vi "temp.vi"   [LabVIEW 2017]
uses:
  Configuration Database/Controls/Congif Data.ctl
  Configuration Database/Controls/Config Commands.ctl
  Error Handler/Controls/Error Type.ctl
  Error Handler/Controls/Error Data.ctl
  Views/Entry Console View/Controls/Entry Console Data.ctl
  Car Wash Controller/Controls/Car Wash States.ctl
  Car Wash Controller/Controls/Vehicle Location.ctl
  Car Wash Controller/Controls/Controller Overhead.ctl
  Car Wash Controller/Controls/CarWash CMD.ctl
  Views/Wash Display Console View/Controls/Car Wash Indicators.ctl
types:
  T1 = typedef "Car Wash Indicators.ctl" = cluster{"Under Body Wash":bool, "Bug Remover":bool, "Pre-Soak":bool, "High Pressure Wash":bool, "Low Pressure Wax":bool, "Spot Free Rinse":bool, "Tire Shine Foam":bool, "Air Dry":bool}
  T2 = typedef "CarWash CMD.ctl" = cluster{"CarWash States":T3, "Variant":variant}
  T3 = typedef "Car Wash States.ctl" = enum16{"Initial", "Wait for start", "Start", "Wait for vehicle", "Wash Step Execution", "Wash Step/Cycle Complete", "Wash Exit", "Wash Abort/Terminate"}
  T4 = typedef "Controller Overhead.ctl" = cluster{"Location change":bool, "Vehicle Location":T5, "CarWash State":T3, "CarWash Next State":T3, "Start change":bool, "Time":dbl, "Elapsed Time":dbl}
  T5 = typedef "Vehicle Location.ctl" = enum16{"Entry", "Station 1", "Station 2", "Station 3", "Exit"}
  T6 = typedef "Car Wash States.ctl" = enum16{"Initial", "Wait for start", "Start", "Wait for vehicle", "Wash Step Execution", "Wash Step Complete", "Wash Cycle Complete", "Wash Exit", "Wash Abort", "Terminate"}
  T7 = typedef "Entry Console Data.ctl" = cluster{"Under Body Wash":bool, "Bug Remover":bool, "Pre-Soak":bool, "High Pressure Wash":bool, "Low Pressure Wax":bool, "Spot Free Rinse":bool, "Tire Shine Foam":bool, "Air Dry":bool}
  T8 = typedef "Error Data.ctl" = cluster{"Error Type":T9, "Error cluster":errorcluster, "Other Data":variant}
  T9 = typedef "Error Type.ctl" = enum16{"Minor Error", "Wash Cycle Error", "System Error", "Other Error"}
  T10 = typedef "Config Commands.ctl" = enum16{"Read records", "Query timing data", "Insert new data records", "Update data records"}
  T11 = typedef "Congif Data.ctl" = cluster{"Wash Step":string, "Station":string, "Step Duration":u32}
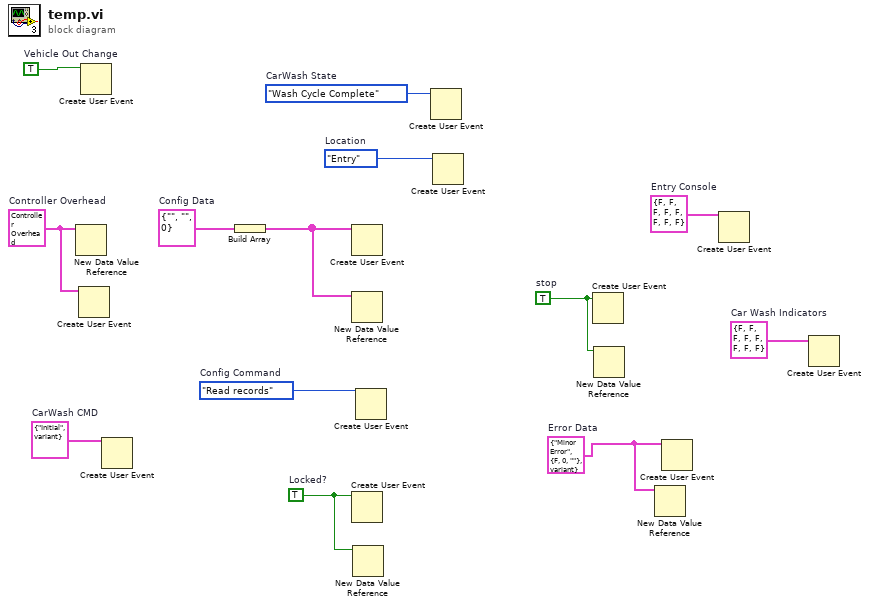
[diagram p0: block diagram]
diagram:
  w1 = T1 {"Under Body Wash"=FALSE, "Bug Remover"=FALSE, "Pre-Soak"=FALSE, "High Pressure Wash"=FALSE, "Low Pressure Wax"=FALSE, "Spot Free Rinse"=FALSE, "Tire Shine Foam"=FALSE, "Air Dry"=FALSE}  # Car Wash Indicators
  w4 = T2 {"CarWash States"=enum."Initial", "Variant"=variant}  # CarWash CMD
  w6 = TRUE  # Vehicle Out Change
  w5 = T4 {"Location change"=FALSE, "Vehicle Location"=enum."Entry", "CarWash State"=enum."Initial", "CarWash Next State"=enum."Initial", "Start change"=FALSE, "Time"=0.0, "Elapsed Time"=0.0}  # Controller Overhead
  w7 = Vehicle_Location."Entry"  # Location
  w8 = Car_Wash_States."Wash Cycle Complete"  # CarWash State
  w9 = T7 {"Under Body Wash"=FALSE, "Bug Remover"=FALSE, "Pre-Soak"=FALSE, "High Pressure Wash"=FALSE, "Low Pressure Wax"=FALSE, "Spot Free Rinse"=FALSE, "Tire Shine Foam"=FALSE, "Air Dry"=FALSE}  # Entry Console
  w10 = T8 {"Error Type"=enum."Minor Error", "Error cluster"={"status"=FALSE, "code"=0, "source"=""}, "Other Data"=variant}  # Error Data
  w11 = TRUE  # stop
  w12 = TRUE  # Locked?
  w13 = Config_Commands."Read records"  # Config Command
  w3 = T11 {"Wash Step"="", "Station"="", "Step Duration"=0}  # Config Data
  n1 = New Data Value Reference(data value=w5) -> ()  [unwired: 1 in, 2 out]
  n2 = Create User Event(user event datatype=w5) -> ()  [unwired: 1 in, 2 out]
  n3 = Create User Event(user event datatype=w6) -> ()  [unwired: 1 in, 2 out]
  n4 = Create User Event(user event datatype=w4) -> ()  [unwired: 1 in, 2 out]
  n5 = Build Array(w3) -> (w2:T11[])
  n6 = Create User Event(user event datatype=w2) -> ()  [unwired: 1 in, 2 out]
  n7 = New Data Value Reference(data value=w2) -> ()  [unwired: 1 in, 2 out]
  n8 = Create User Event(user event datatype=w12) -> ()  [unwired: 1 in, 2 out]
  n9 = New Data Value Reference(data value=w12) -> ()  [unwired: 1 in, 2 out]
  n10 = Create User Event(user event datatype=w13) -> ()  [unwired: 1 in, 2 out]
  n11 = Create User Event(user event datatype=w8) -> ()  [unwired: 1 in, 2 out]
  n12 = Create User Event(user event datatype=w7) -> ()  [unwired: 1 in, 2 out]
  n13 = Create User Event(user event datatype=w11) -> ()  [unwired: 1 in, 2 out]
  n14 = New Data Value Reference(data value=w11) -> ()  [unwired: 1 in, 2 out]
  n15 = New Data Value Reference(data value=w10) -> ()  [unwired: 1 in, 2 out]
  n16 = Create User Event(user event datatype=w10) -> ()  [unwired: 1 in, 2 out]
  n17 = Create User Event(user event datatype=w9) -> ()  [unwired: 1 in, 2 out]
  n18 = Create User Event(user event datatype=w1) -> ()  [unwired: 1 in, 2 out]
